vi "test.vi"() -> ()   [LabVIEW 2013]
uses:
  shared programs/GUI_Template/GUI_master/tcp_new_data_event.ctl
  shared programs/GUI_Template/GUI_master/tcp new data cluster.ctl
  <vilib>/vision/Image Controls.llb/IMAQ Image.ctl
panel:
  in  "Target.X::1":dbl=200.0 caption="Target X" format="%#.2p"
  in  "Target.Y::1":dbl=200.0 caption="Target Y" format="%#.2p"
  in  "stop":bool
  out "image::1":T1(plugin-control) caption="StagingM1Near"
  out "tcp data event":T2
  out "error IO 2":errorcluster
  in  "GUIdevice 1":string="StagingM1Near"
  in  "insert tag":bool=TRUE
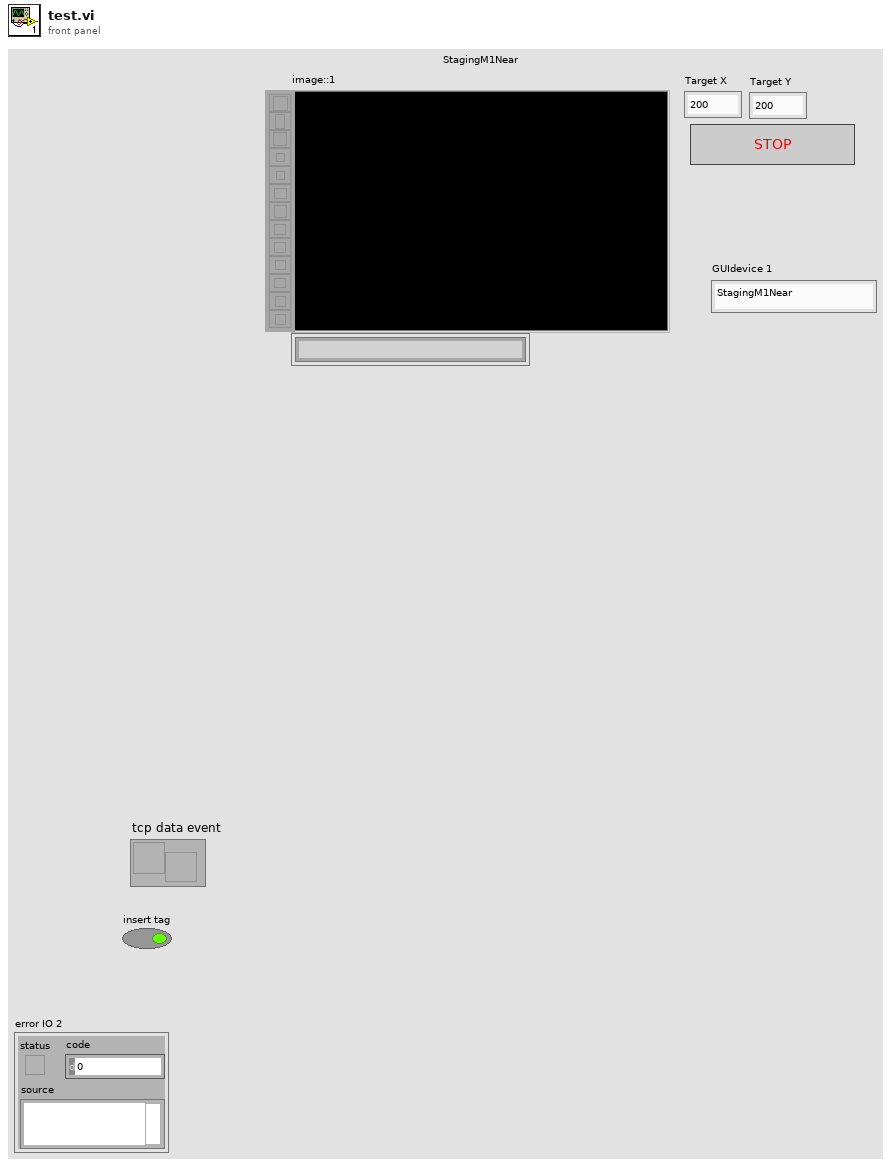
[diagram p1: front panel]
types:
  T1 = typedef "IMAQ Image.ctl" = refnum<image>
  T2 = typedef "tcp_new_data_event.ctl" = refnum<user-event>
  T3 = typedef "tcp new data cluster.ctl" = cluster{"EventEnum":enum16{"new data", "connection status update"}, "Device name":string}
  T4 = typedef "ROI Descriptor" = cluster{"Global Rectangle":i32[], "Contours":cluster{"ID":enum32{"External", "Internal"}, "Type":u32, "Coordinates":i32[]}[]}
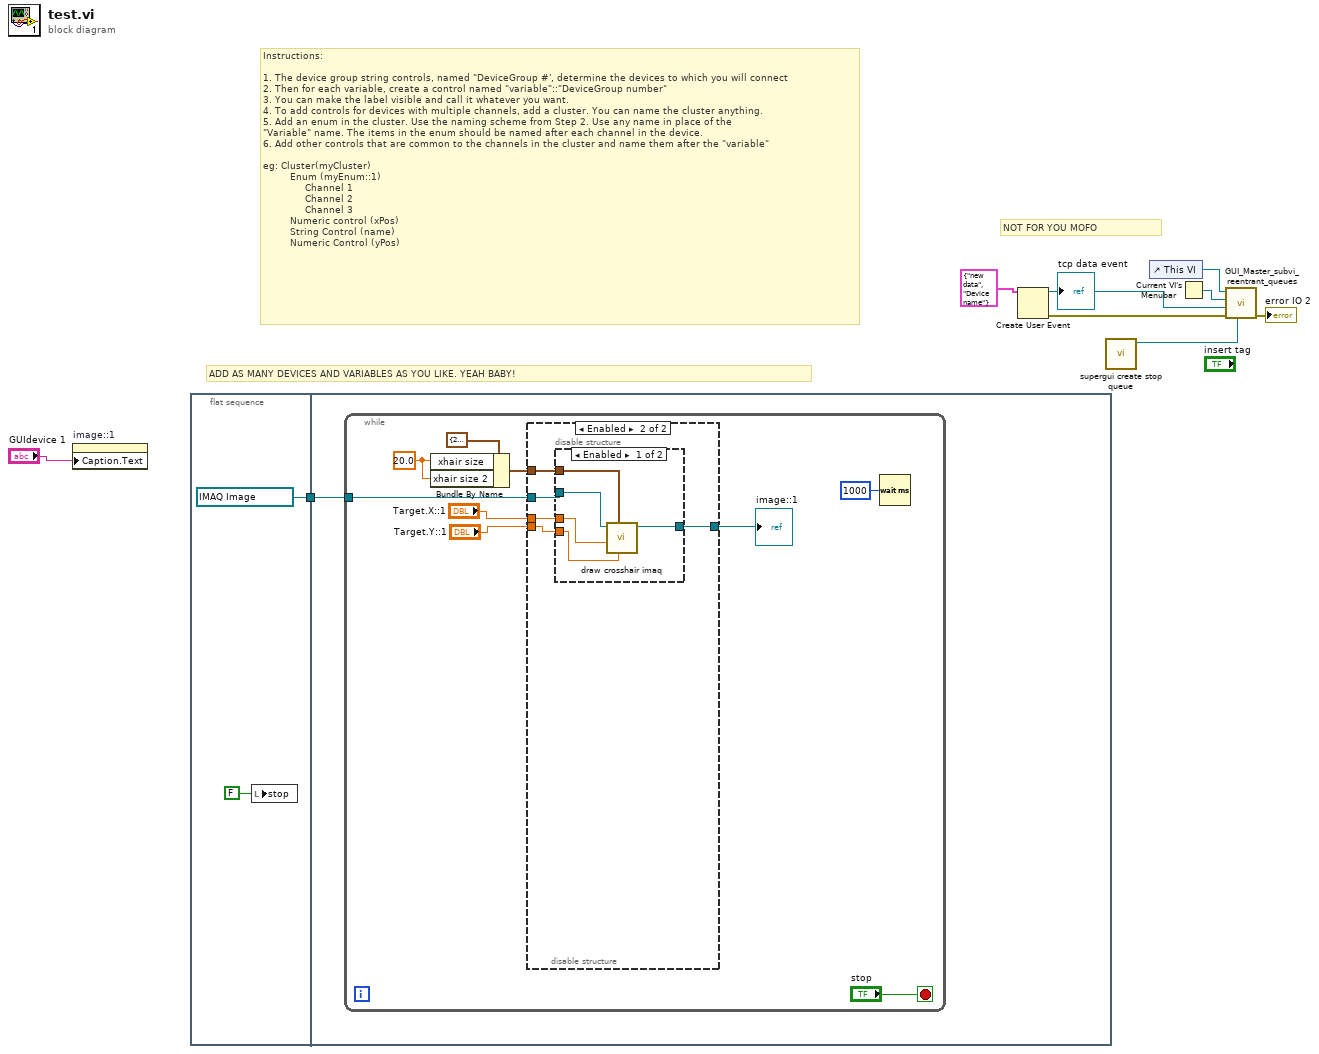
[diagram p0: block diagram]
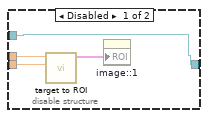
[diagram p2: hidden frame]
diagram:
  # "Instructions:\n\n1. The device group string controls, named \"DeviceGroup #', determine the devices to which you will connect\n2. Then for each variable, create a control named \"variable\"::\"DeviceGroup number\"\n3. You can make the label visible and call it whatever you want.\n4. To add controls for devices with multiple channels, add a cluster. You can name the cluster anything.\n5. Add an enum in the cluster. Use the naming scheme from Step 2. Use any name in place of the \n\"Variable\" name. The items in the enum should be named after each channel in the device. \n6. Add other controls that are common to the channels in the cluster and name them after the \"variable\"\n\neg: Cluster(myCluster)\n         Enum (myEnum::1)\n              Channel 1 \n              Channel 2\n              Channel 3\n         Numeric control (xPos)\n         String Control (name)\n         Numeric Control (yPos)"
  # "ADD AS MANY DEVICES AND VARIABLES AS YOU LIKE. YEAH BABY!"
  # "NOT FOR YOU MOFO"
  n1 = property on="image::1" class="ImageControl"("Caption.Text"="GUIdevice 1") -> ()  [unwired: 2 in, 2 out]
  n2 = flat-sequence {
    tunnel: [T1 refnum ("New Image")] -> w9
    tunnel: w9 -> [w12]
    frame #0 {
      n3 = local write "stop"(FALSE ("stop")) -> ()
    }
    frame #1 {
      n4 = while {
        tunnel: w12 -> [w17]
        stop <- "stop" stop-if-true
        w14 = 20.0 ("size")
        n5 = Bundle By Name(cluster=cluster{"xhair size":dbl, "xhair size 2":dbl} {"xhair size"=20.0, "xhair size 2"=20.0} ("size"), "xhair size"=w14, "xhair size 2"=w14) -> (w13:cluster{"xhair size":dbl, "xhair size 2":dbl})
        n6 = disable-structure shown="Enabled" {
          disable-tunnel: "Target.X::1" -> [w25 w30]
          disable-tunnel: "Target.Y::1" -> [w24 w29]
          disable-tunnel: w17 -> [w22 w28]
          disable-tunnel: [w22 w27] -> w16
          disable-tunnel: w13 -> [_ w26]
          frame Disabled {
            n7 = call "target to ROI.vi"("Target.Y::1"=w24, "Target.X::1"=w25) -> ("ROI Descriptor out"=w23:T4)  [unwired: 9 in]
            n8 = property on="image::1" class="ImageControl"("ROI"=w23) -> ()  [unwired: 2 in, 2 out]
          }
          frame Enabled {
            n9 = disable-structure shown="Enabled" {
              disable-tunnel: w30 -> [w35 _]
              disable-tunnel: w29 -> [w34 _]
              disable-tunnel: w28 -> [w33 w36]
              disable-tunnel: [w32 w36] -> w27
              disable-tunnel: w26 -> [w31 _]
              frame Enabled {
                n10 = call "draw crosshair imaq.vi"("Target.Y"=w34, "size"=w31, "Target.X"=w35, "image in"=w33) -> ("image out"=w32:T1)  [unwired: 6 in, 1 out]
              }
              frame Disabled {
              }
            }
          }
        }
        "image::1" <- w16
        n11 = Wait (ms)(milliseconds to wait=u32 1000) -> ()  [unwired: 1 out]
      }
    }
  }
  n12 = Create User Event(user event datatype=T3 {"EventEnum"=enum."new data", "Device name"="Device name"} ("New Event")) -> (user event=w3:refnum<user-event>, error out=w4:errorcluster)  [unwired: 1 in]
  "tcp data event" <- w3
  n13 = call "supergui create stop queue.vi"() -> ("STOP Queue out"=w1:refnum<queue>)  [unwired: 11 in]
  n14 = control-ref of="This VI"() -> (w7:refnum<vi>)
  n15 = Current VI's Menubar() -> (w6:refnum<k9>)
  n16 = call "GUI_Master_subvi_reentrant_queues.vi"("STOP Queue in"=w1, "error in (no error)"=w4, "tcp data event"=w3, "Caller menu reference"=w6, "Caller VI ref"=w7) -> ("error out"=→"error IO 2":errorcluster)  [unwired: 6 in]
